vi "Get Joystick.vi"() -> (2 "Robot Controls":T1)   [LabVIEW 2016]
uses:
  Robot Controls.ctl
  <vilib>/Rock Robotics/WPI/Utilities/WPI_GetSetVariantRefNum.vi
panel:
  in  "Robot Controls":T1
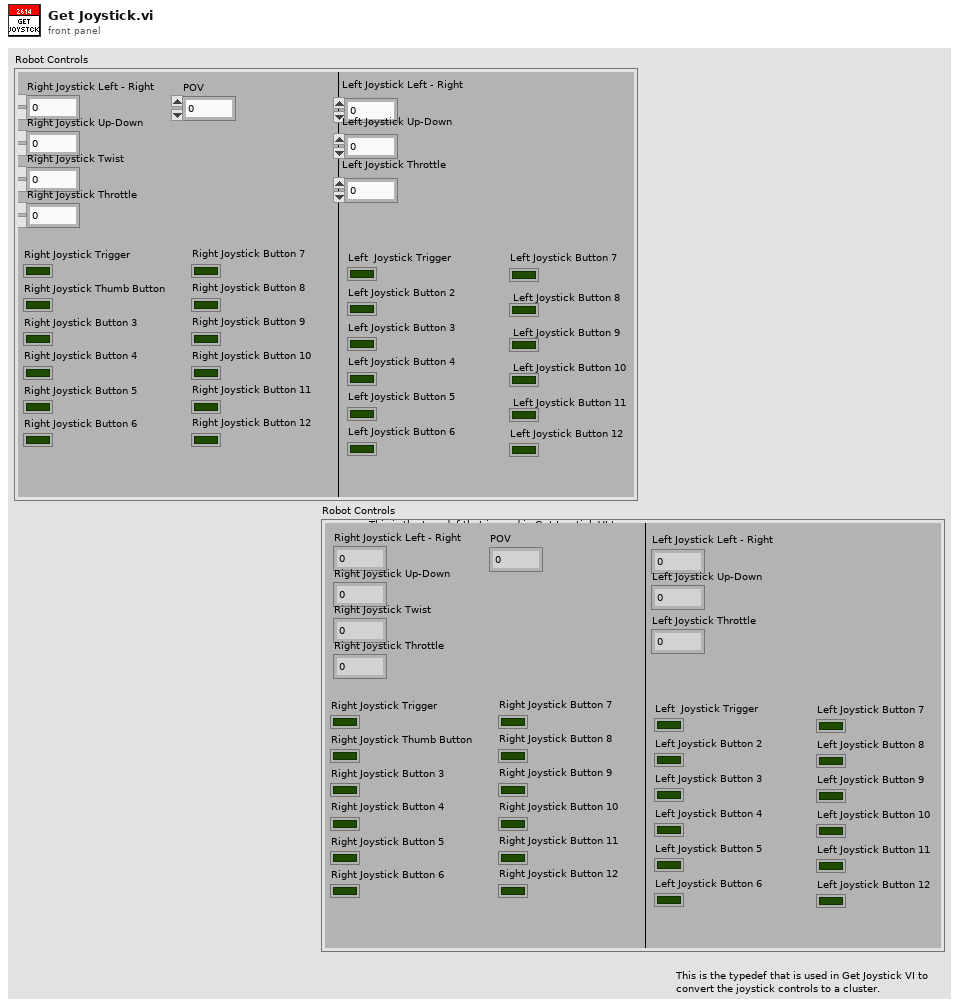
[diagram p1: front panel]
types:
  T1 = typedef "Robot Controls.ctl" = cluster{"Right Joystick Trigger":bool, "Right Joystick Thumb Button":bool, "Right Joystick Button 3":bool, "Right Joystick Button 4":bool, "Right Joystick Button 5":bool, "Right Joystick Button 7":bool, "Right Joystick Button 8":bool, "Right Joystick Button 9":bool, "Right Joystick Button 10":bool, "Right Joystick Button 11":bool, "Right Joystick Left - Right":dbl, "Right Joystick Up-Down":dbl, "Right Joystick Twist":dbl, "Right Joystick Throttle":dbl, "Right Joystick Button 6":bool, "Right Joystick Button 12":bool, "Left  Joystick Trigger":bool, "Left Joystick Button 2":bool, "Left Joystick Button 3":bool, "Left Joystick Left - Right":dbl, "Left Joystick Up-Down":dbl, "Left Joystick Throttle ":dbl, "Left Joystick Button 4":bool, "Left Joystick Button 5":bool, "Left Joystick Button 6":bool, "Left Joystick Button 7":bool, "Left Joystick Button 8":bool, "Left Joystick Button 9":bool, "Left Joystick Button 10":bool, "Left Joystick Button 11":bool, "Left Joystick Button 12":bool, "POV":dbl}
  T2 = typedef "WPI_JoystickDevRef.ctl" = cluster{"Device":T3}
  T3 = typedef "WPI_JoystickDeviceEnum.ctl" = enum16{"USB 0", "USB 1", "USB 2", "USB 3", "USB 4", "USB 5"}
  T4 = cluster{"Axes[0]":dbl, "Axes[1]":dbl, "Axes[2]":dbl, "Axes[3]":dbl, "Axes[4]":dbl, "Axes[5]":dbl, "Axes[6]":dbl, "Axes[7]":dbl, "Axes[8]":dbl}
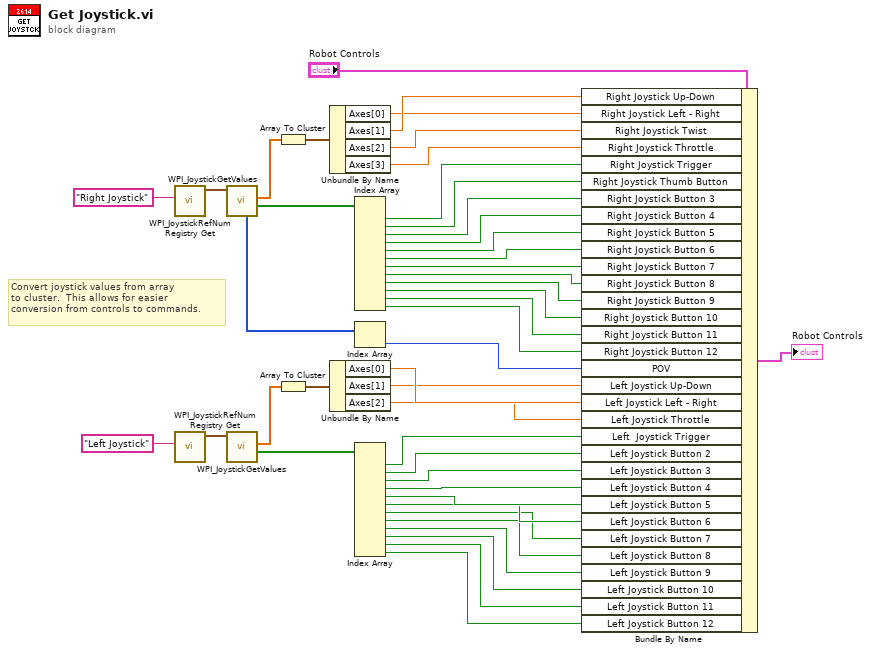
[diagram p0: block diagram]
diagram:
  # "Convert joystick values from array \nto cluster.  This allows for easier\nconversion from controls to commands."
  n1 = call <vilib>:"WPI_JoystickRefNum Registry Get.vi"("refnum name"="Right Joystick") -> ("JoystickDevRef"=w44:T2)  [unwired: 9 in, 1 out]
  n2 = call <vilib>:"WPI_JoystickRefNum Registry Get.vi"("refnum name"="Left Joystick") -> ("JoystickDevRef"=w38:T2)  [unwired: 9 in, 1 out]
  n3 = call <vilib>:"WPI_JoystickGetValues.vi"("JoystickDevRef"=w44) -> ("Buttons"=w40:bool[], "Axes"=w43:dbl[], "POVs"=w2:i16[])  [unwired: 6 in, 2 out]
  n4 = call <vilib>:"WPI_JoystickGetValues.vi"("JoystickDevRef"=w38) -> ("Buttons"=w35:bool[], "Axes"=w37:dbl[])  [unwired: 6 in, 3 out]
  n5 = Array To Cluster(array=w43) -> (cluster=w42:T4)
  n6 = Array To Cluster(array=w37) -> (cluster=w36:T4)
  n7 = Unbundle By Name(w42) -> ("Axes[0]"=w31:dbl, "Axes[1]"=w32:dbl, "Axes[2]"=w34:dbl, "Axes[3]"=w33:dbl)
  n8 = Unbundle By Name(w36) -> ("Axes[0]"=w30:dbl, "Axes[1]"=w29:dbl, "Axes[2]"=w28:dbl)
  n9 = Index Array(array=w40) -> (element #1=w27:bool, element #2=w26:bool, element #3=w25:bool, element #4=w24:bool, element #5=w23:bool, element #6=w22:bool, element #7=w21:bool, element #8=w20:bool, element #9=w19:bool, element #10=w18:bool, element #11=w17:bool, element #12=w16:bool)  [unwired: 12 in]
  n10 = Index Array(array=w2) -> (element=w1:i16)  [unwired: 1 in]
  n11 = Index Array(array=w35) -> (element #1=w15:bool, element #2=w14:bool, element #3=w13:bool, element #4=w12:bool, element #5=w11:bool, element #6=w10:bool, element #7=w9:bool, element #8=w8:bool, element #9=w7:bool, element #10=w6:bool, element #11=w5:bool, element #12=w4:bool)  [unwired: 12 in]
  n12 = Bundle By Name(cluster="Robot Controls", "Right Joystick Up-Down"=w32, "Right Joystick Left - Right"=w31, "Right Joystick Twist"=w34, "Right Joystick Throttle"=w33, "Right Joystick Trigger"=w27, "Right Joystick Thumb Button"=w26, "Right Joystick Button 3"=w25, "Right Joystick Button 4"=w24, "Right Joystick Button 5"=w23, "Right Joystick Button 6"=w22, "Right Joystick Button 7"=w21, "Right Joystick Button 8"=w20, "Right Joystick Button 9"=w19, "Right Joystick Button 10"=w18, "Right Joystick Button 11"=w17, "Right Joystick Button 12"=w16, "POV"=w1, "Left Joystick Up-Down"=w29, "Left Joystick Left - Right"=w30, "Left Joystick Throttle"=w28, "Left  Joystick Trigger"=w15, "Left Joystick Button 2"=w14, "Left Joystick Button 3"=w13, "Left Joystick Button 4"=w12, "Left Joystick Button 5"=w11, "Left Joystick Button 6"=w10, "Left Joystick Button 7"=w9, "Left Joystick Button 8"=w8, "Left Joystick Button 9"=w7, "Left Joystick Button 10"=w6, "Left Joystick Button 11"=w5, "Left Joystick Button 12"=w4) -> (→"Robot Controls":T1)
